vi "Write States.vi"(8 "error in (no error)":errorcluster, 10 "States":T1, 11 "BallPlacementEnemyTactic in":refnum<class "BallPlacementEnemyTactic.lvclass">) -> (0 "error out":errorcluster, 3 "BallPlacementEnemyTactic out":refnum<class "BallPlacementEnemyTactic.lvclass">)   [LabVIEW 2020, in "BallPlacementEnemyTactic.lvclass"]
uses:
  BallPlacementEnemyTactic.lvclass
  StatesBallPlacementEnemyTactic.ctl
  BallPlacementEnemyTactic.lvclass/BallPlacementEnemyTactic.ctl
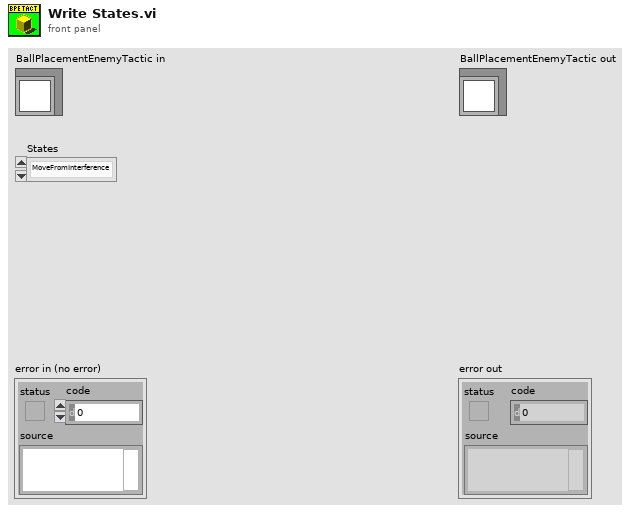
[diagram p1: front panel]
types:
  T1 = typedef "BallPlacementEnemyTactic.lvclass/StatesBallPlacementEnemyTactic.ctl" = enum16{"MoveFromInterference", "Halt", "Exit"}
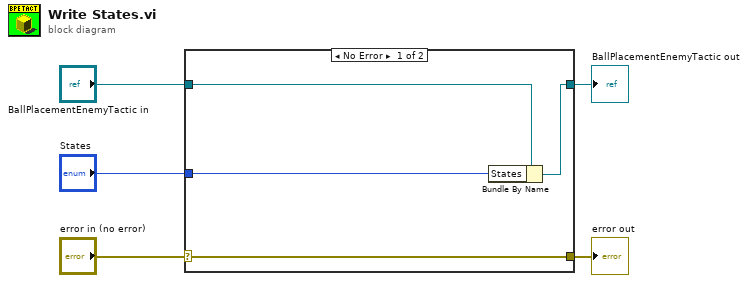
[diagram p0: block diagram]
diagram:
  n1 = case shown="No Error" "error in (no error)" {
    selector: "error in (no error)" -> [w9 w10]
    tunnel: [w9 w10] -> w4
    tunnel: [w7 w11] -> w2
    tunnel: "BallPlacementEnemyTactic in" -> [w8 w11]
    tunnel: "States" -> [w6 _]
    frame No Error {
      n2 = Bundle By Name(cluster=w8, "States"=w6) -> (w7:refnum<class "BallPlacementEnemyTactic.lvclass">)
    }
    frame Error {
    }
  }
  "error out" <- w4
  "BallPlacementEnemyTactic out" <- w2
